vi "PreconfiguredSleeveData.vi"() -> ()   [LabVIEW 2013]
panel:
  in  "PreconfiguredSleeveData":T1
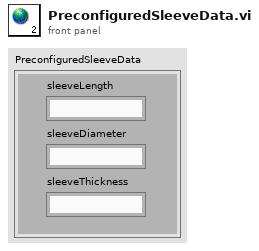
[diagram p1: front panel]
types:
  T1 = cluster{"sleeveLength":string, "sleeveDiameter":string, "sleeveThickness":string}
diagram:
